vi "Find File ID.vi"(10 "File ID":i32, 11 "File List":T1[](array[typedef])) -> (1 "Array Index":i32, 2 "Found?":bool, 3 "File Info":T1)   [LabVIEW 2020, in "Peer Review.lvclass"]
uses:
  Peer Review.lvclass
  TypeDefs/File Info.ctl
  TypeDefs/File State.ctl
  TypeDefs/VI Type.ctl
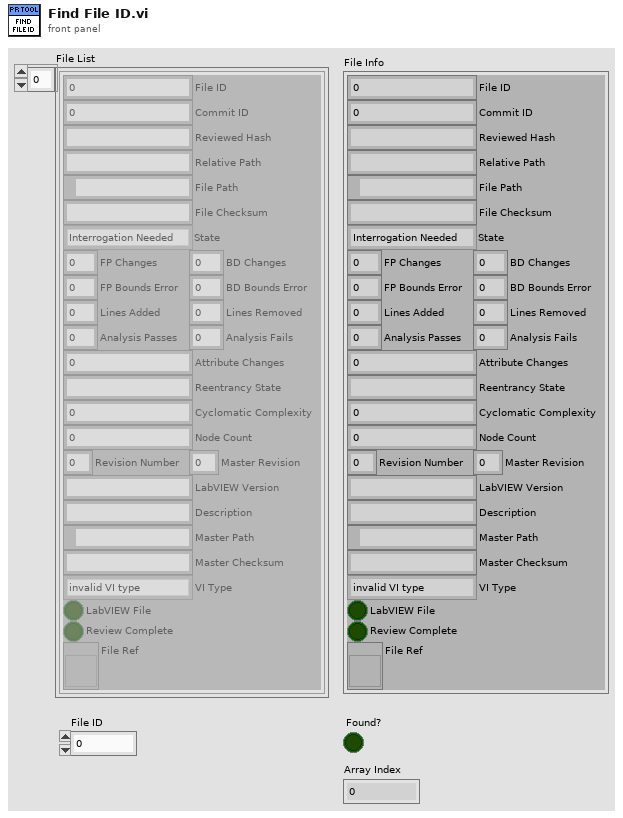
[diagram p1: front panel]
types:
  T1 = typedef "Peer Review.lvclass/File Info.ctl" = cluster{"File ID":i32, "Commit ID":i32, "Reviewed Hash":string, "Relative Path":string, "File Path":path, "File Checksum":string, "State":T2, "FP Changes":i32, "BD Changes":i32, "FP Bounds Error":dbl, "BD Bounds Error":dbl, "Lines Added":i32, "Lines Removed":i32, "Analysis Passes":i32, "Analysis Fails":i32, "Attribute Changes":i32, "Reentrancy State":string, "Cyclomatic Complexity":i32, "Node Count":i32, "Revision Number":u32, "LabVIEW Version":string, "Description":string, "Master Path":path, "Master Checksum":string, "VI Type":T3, "LabVIEW File":bool, "Review Complete":bool, "File Ref":refnum<vi>, "Master Revision":u32}
  T2 = typedef "Peer Review.lvclass/File State.ctl" = enum16{"Interrogation Needed", "Modified", "Deleted", "Added", "Matches Previous", "No Changes", "Moved", "Empty File"}
  T3 = typedef "Peer Review.lvclass/VI Type.ctl" = enum32{"invalid VI type", "Standard VI", "Control VI", "Global VI", "Polymorphic VI", "Configuration VI", "SubSystem", "Facade VI", "Method VI", "Statechart Diagram VI"}
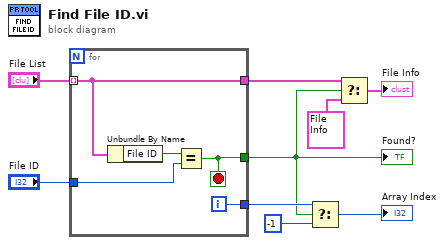
[diagram p0: block diagram]
diagram:
  n1 = for {
    tunnel: "File List" -> [w11] mode=indexing
    tunnel: "File ID" -> [w14]
    tunnel: [w12] -> w4
    tunnel: [w11] -> w3
    tunnel: [w10] -> w7
    i -> [w10]
    stop <- w12 stop-if-true
    n2 = Unbundle By Name(w11) -> ("File ID"=w13:i32)
    n3 = Equal?(x=w13, y=w14) -> (x = y?=w12:bool)
  }
  "Found?" <- w4
  n4 = Select(t=w7, s=w4, f=-1) -> (s? t:f=→"Array Index":i32)
  n5 = Select(t=w3, s=w4, f=T1 {"File ID"=0, "Commit ID"=0, "Reviewed Hash"="", "Relative Path"="", "File Path"=path "", "File Checksum"="", "State"=enum."Interrogation Needed", "FP Changes"=0, "BD Changes"=0, "FP Bounds Error"=0.0, "BD Bounds Error"=0.0, "Lines Added"=0, "Lines Removed"=0, "Analysis Passes"=0, "Analysis Fails"=0, "Attribute Changes"=0, "Reentrancy State"="", "Cyclomatic Complexity"=0, "Node Count"=0, "Revision Number"=0, "LabVIEW Version"="", "Description"="", "Master Path"=path "", "Master Checksum"="", "VI Type"=enum."invalid VI type", "LabVIEW File"=FALSE, "Review Complete"=FALSE, "File Ref"=refnum, "Master Revision"=0}) -> (s? t:f=→"File Info":T1)
